vi "Autonomous Independent.vi"() -> ()   [LabVIEW 2015]
doc: "This VI is called when autonomous begins, and will automatically be terminated when autonomous ends. You can carry out timed or sensor driven robot movement independently without needing to return to the caller."
uses:
  <vilib>/Rock Robotics/WPI/Utilities/WPI_GetSetVariantRefNum.vi
  <vilib>/Rock Robotics/Network Tables/NT Write Numeric Array.vi
  <vilib>/Rock Robotics/Network Tables/NT Read Boolean.vi
  <vilib>/Rock Robotics/Network Tables/NT Write Boolean.vi
  <vilib>/Rock Robotics/Network Tables/NT Write Number.vi
  <vilib>/Rock Robotics/Network Tables/NT Read Number.vi
  <vilib>/Rock Robotics/WPI/RobotDrive/WPI_RobotDriveArcadeDrive_Standard(NoSaturation).vi
panel:
  out "Low Switch":bool
  out "High Switch":bool
  out "POT Sensor Meter":dbl(knob) scale=78.0..98.0
  out "POT Sensor Value":dbl
  # "Be sure to right-click and choose Data Operations>>Make Current Value default if you want to save the array values with the VI"
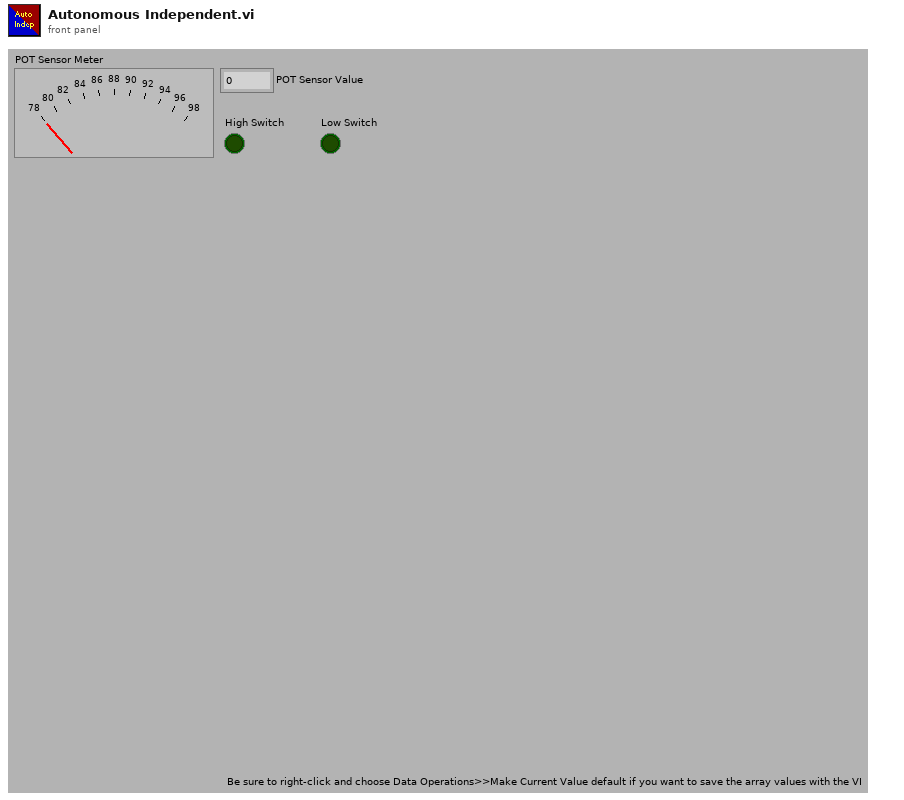
[diagram p1: front panel]
types:
  T1 = typedef "WPI_JoystickDevRef.ctl" = cluster{"Device":T2}
  T2 = typedef "WPI_JoystickDeviceEnum.ctl" = enum16{"USB 0", "USB 1", "USB 2", "USB 3", "USB 4", "USB 5"}
  T3 = typedef "WPI_SwitchDevRef.ctl" = cluster{"DevStatus":errorcluster, "DIO Channel":T4, "CntIndex":T5, "Normally Closed":bool}
  T4 = typedef "FPGA_DIOChannel.ctl" = enum8{"DIO 0", "DIO 1", "DIO 2", "DIO 3", "DIO 4", "DIO 5", "DIO 6", "DIO 7", "DIO 8", "DIO 9", "DIO MXP 0", "DIO MXP 1", "DIO MXP 2", "DIO MXP 3", "DIO MXP 4", "DIO MXP 5", "DIO MXP 6", "DIO MXP 7", "DIO MXP 8", "DIO MXP 9", "DIO MXP 10", "DIO MXP 11", "DIO MXP 12", "DIO MXP 13", "DIO MXP 14", "DIO MXP 15", "Invalid"}
  T5 = typedef "FPGA_CounterCtrSystemIndex.ctl" = enum8{"Ctr 0", "Ctr 1", "Ctr 2", "Ctr 3", "Ctr 4", "Ctr 5", "Ctr 6", "Ctr 7", "Invalid"}
  T6 = typedef "WPI_PotentiometerDevRef.ctl" = cluster{"DevStatus":errorcluster, "Analog Channel":T7, "Invert Output":bool}
  T7 = typedef "FPGA_AIChannel.ctl" = enum8{"AI 0", "AI 1", "AI 2", "AI 3", "AI MXP 0", "AI MXP 1", "AI MXP 2", "AI MXP 3", "Invalid"}
  T8 = typedef "WPI_MotorControlDeviceRef.ctl" = cluster{"DeviceStatus":errorcluster, "Type":T9, "PWM":cluster{"PWM Channel":T10, "DeadBand":T11}, "CAN":cluster{"Device Number":u8, "Control Mode":T12, "Semaphore":T13, "Max Vout":dbl, "TalonSRX Control Mode":T14}, "Invert":bool}
  T9 = typedef "WPI_MotorControlType.ctl" = enum16{"PWM", "CAN", "CANTalonSRX"}
  T10 = typedef "FPGA_DIOPWMChannel.ctl" = enum8{"PWM 0", "PWM 1", "PWM 2", "PWM 3", "PWM 4", "PWM 5", "PWM 6", "PWM 7", "PWM 8", "PWM 9", "PWM MXP 0", "PWM MXP 1", "PWM MXP 2", "PWM MXP 3", "PWM MXP 4", "PWM MXP 5", "PWM MXP 6", "PWM MXP 7", "PWM MXP 8", "PWM MXP 9", "Invalid"}
  T11 = typedef "WPI_PWMDeadband.ctl" = cluster{"Name":string, "maxPositivePwm":i32, "minPositivePwm":i32, "centerPwm":i32, "maxNegativePwm":i32, "minNegativePwm":i32, "angularRange":u16}
  T12 = typedef "WPI_CANJaguar_ControlMode.ctl" = enum8{"Percent VBus", "Current", "Speed", "Position", "Voltage"}
  T13 = typedef "Semaphore RefNum" = refnum<k1>
  T14 = typedef "WPI_CANTalonSRX_APIControlMode.ctl" = enum8{"Percent VBus", "Speed", "Position", "Slave", "Unchanged / Invalid", "Voltage Compensation", "Current", "Motion Profile"}
  T15 = typedef "WPI_RobotDriveDevRef.ctl" = cluster{"DevStatus":errorcluster, "Motors[]":T8[], "Square Inputs":bool, "Max Output":dbl}
  T16 = typedef "WPI_CounterDevRef.ctl" = cluster{"DevStatus":errorcluster, "CntIndex":T5}
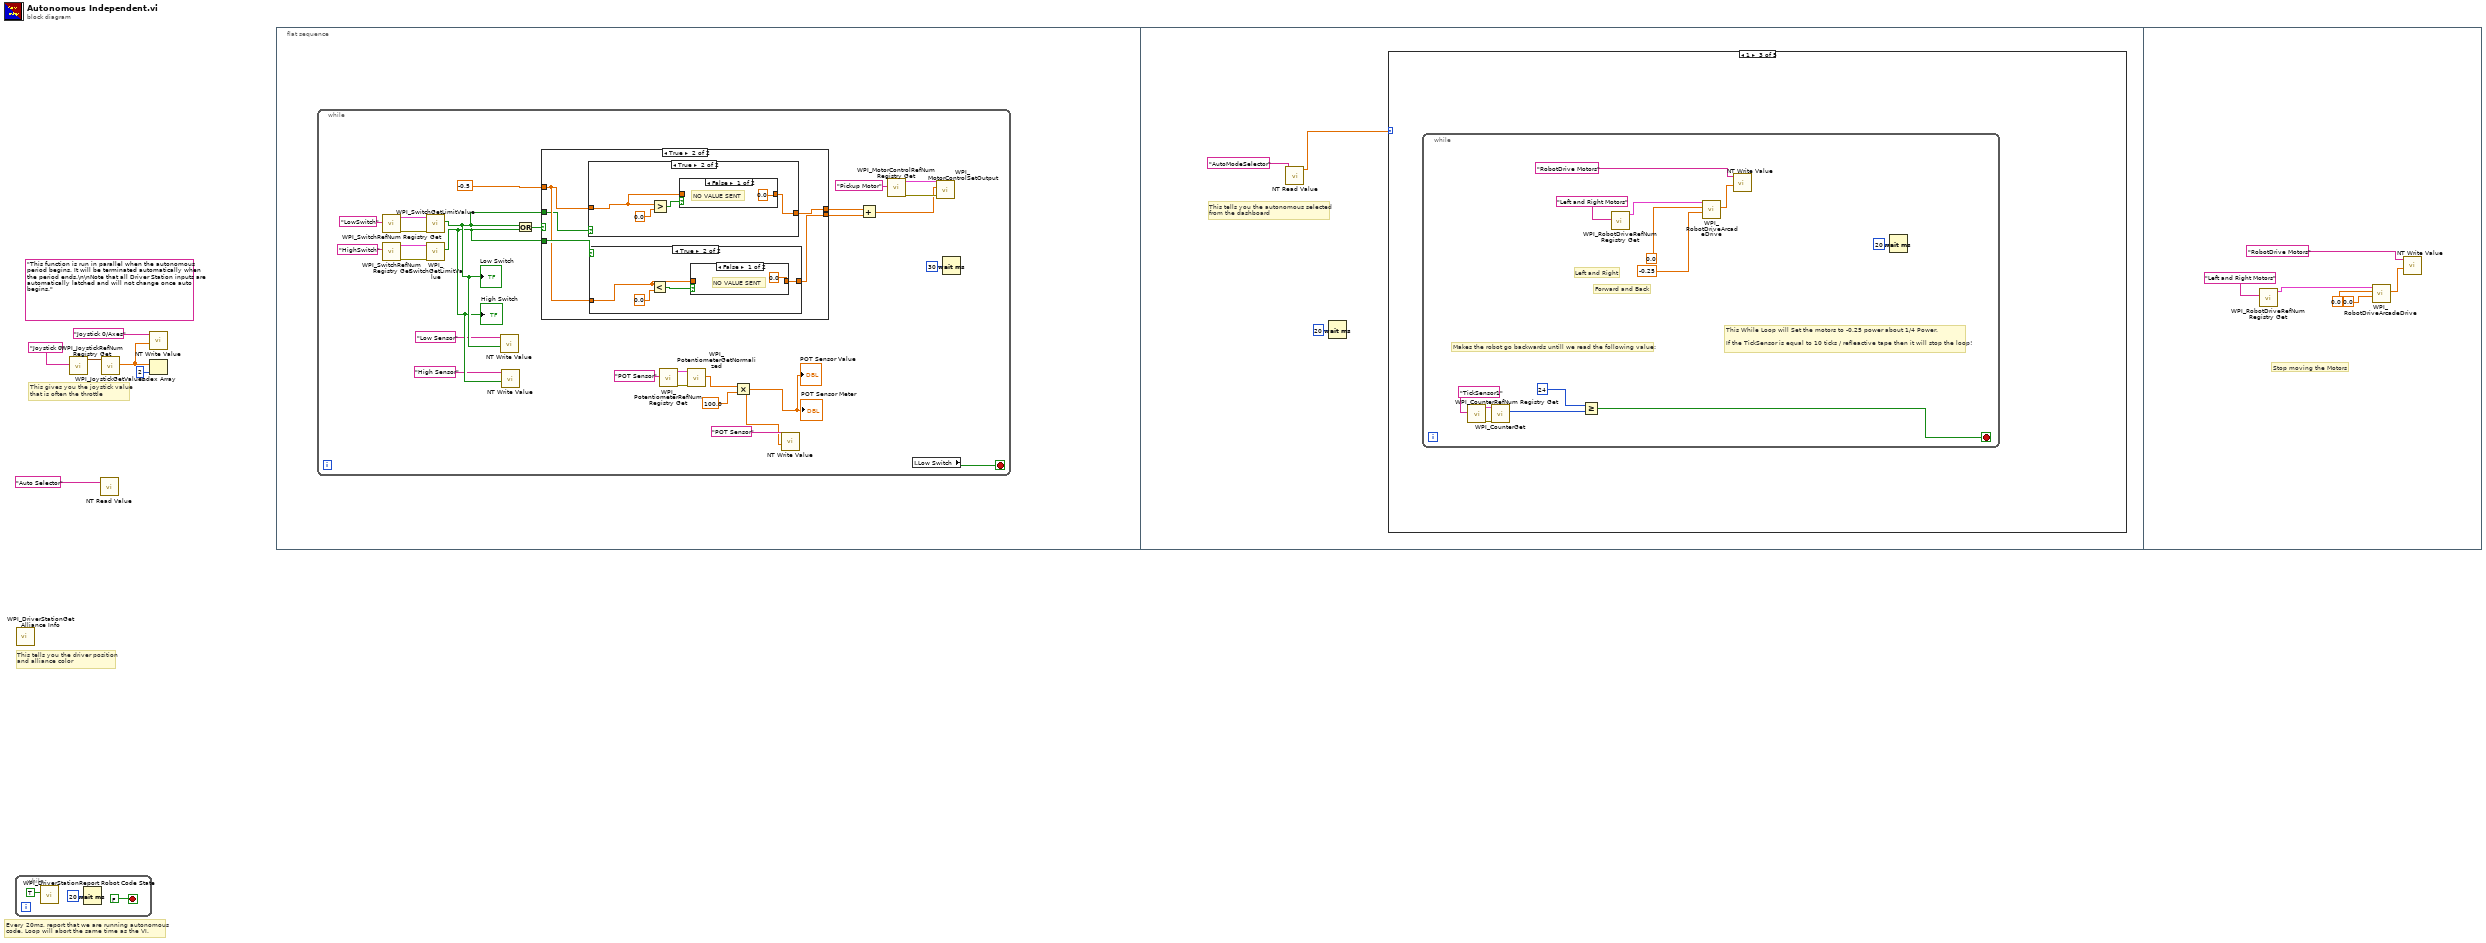
[diagram p0: block diagram]
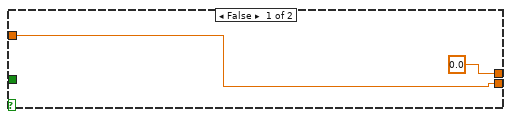
[diagram p2: hidden frame]
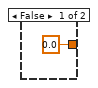
[diagram p3: hidden frame]
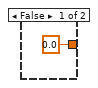
[diagram p5: hidden frame]
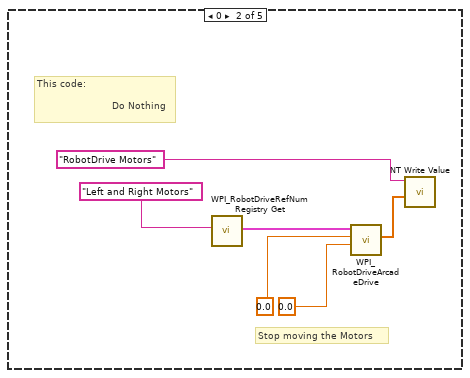
[diagram p8: hidden frame]
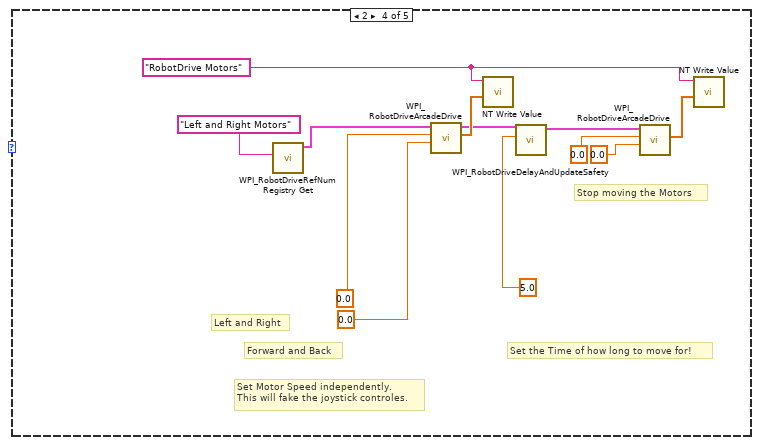
[diagram p9: hidden frame]
diagram:
  (unwired) "This function is run in parallel when the autonomous period begins. It will be terminated automatically when the period ends.\n\nNote that all Driver Station inputs are automatically latched and will not change once auto begins."
  # "Every 20ms, report that we are running autonomous\ncode. Loop will abort the same time as the VI."
  # "This gives you the joystick value\nthat is often the throttle"
  # "This tells you the driver position\nand alliance color"
  n1 = while {
    stop <- FALSE stop-if-true
    n2 = call <vilib>:"WPI_DriverStationReport Robot Code State.vi"("Autonomous"=TRUE) -> ()  [unwired: 10 in, 1 out]
    n3 = Wait (ms)(milliseconds to wait=u32 20) -> ()  [unwired: 1 out]
  }
  n4 = call <vilib>:"WPI_DriverStationGet Alliance Info.vi"() -> ()  [unwired: 12 out]
  n5 = call <vilib>:"WPI_JoystickRefNum Registry Get.vi"("refnum name"="Joystick 0") -> ("JoystickDevRef"=w5:T1)  [unwired: 1 in, 9 out]
  n6 = call-poly <vilib>:"NT Read Value.vi"("Name"="Auto Selector") -> ()  [unwired: 9 in, 2 out]
  n7 = call <vilib>:"WPI_JoystickGetValues.vi"("JoystickDevRef"=w5) -> ("Axes"=w3:dbl[])  [unwired: 6 in, 4 out]
  n8 = call-poly <vilib>:"NT Write Value.vi"("Numeric Array"=w3, "Name"="Joystick 0/Axes") -> ()  [unwired: 9 in, 1 out]
  n9 = Index Array(array=w3, index=2) -> ()  [unwired: 1 out]
  n10 = flat-sequence {
    frame #0 {
      n11 = while {
        stop <- w11 stop-if-true
        n12 = call <vilib>:"WPI_SwitchRefNum Registry Get.vi"("refnum name"="LowSwitch") -> ("error out"=w34:errorcluster, "SwitchDevRef"=w35:T3)  [unwired: 9 in]
        n13 = call <vilib>:"WPI_SwitchRefNum Registry Get.vi"("refnum name"="HighSwitch") -> ("error out"=w31:errorcluster, "SwitchDevRef"=w32:T3)  [unwired: 9 in]
        n14 = call <vilib>:"WPI_SwitchGetLimitValue.vi"("error in (no error)"=w34, "SwitchDevRef"=w35) -> ("Switch Pressed"=w19:bool)  [unwired: 7 in, 2 out]
        "Low Switch" <- w19
        n15 = call <vilib>:"WPI_SwitchGetLimitValue.vi"("error in (no error)"=w31, "SwitchDevRef"=w32) -> ("Switch Pressed"=w18:bool)  [unwired: 7 in, 2 out]
        "High Switch" <- w18
        n16 = call-poly <vilib>:"NT Write Value.vi"("Boolean"=w19, "Name"="Low Sensor") -> ()  [unwired: 9 in, 1 out]
        n17 = call-poly <vilib>:"NT Write Value.vi"("Boolean"=w18, "Name"="High Sensor") -> ()  [unwired: 9 in, 1 out]
        n18 = Or(x=w19, y=w18) -> (x .or. y?=w36:bool)
        n19 = case shown="True" w36 {
          tunnel: w19 -> [_ w41]
          tunnel: w18 -> [_ w43]
          tunnel: -0.5 ("Axes[1]") -> [w37 w42]
          tunnel: [0.0 ("Axes[1]") w40] -> w25
          tunnel: [w37 w39] -> w24
          frame False {
          }
          frame True {
            n20 = case shown="True" w41 {
              tunnel: w42 -> [_ w53]
              tunnel: [0.0 ("Axes[1]") w52] -> w40
              frame False {
              }
              frame True {
                n21 = Greater?(x=w53, y=0.0) -> (0:w54:bool)
                n22 = case shown="False" w54 {
                  tunnel: [0.0 ("Axes[1]") w57] -> w52
                  tunnel: w53 -> [_ w57]
                  frame False {
                    # "NO VALUE SENT"
                  }
                  frame True {
                  }
                }
              }
            }
            n23 = case shown="True" w43 {
              tunnel: w42 -> [_ w45]
              tunnel: [0.0 ("Axes[1]") w46] -> w39
              frame False {
              }
              frame True {
                n24 = Less?(x=w45, y=0.0) -> (x < y?=w47:bool)
                n25 = case shown="False" w47 {
                  tunnel: [0.0 ("Axes[1]") w50] -> w46
                  tunnel: w45 -> [_ w50]
                  frame False {
                    # "NO VALUE SENT"
                  }
                  frame True {
                  }
                }
              }
            }
          }
        }
        n26 = call <vilib>:"WPI_PotentiometerRefNum Registry Get.vi"("refnum name"="POT Sensor") -> ("error out"=w23:errorcluster, "PotDevRef"=w22:T6)  [unwired: 9 in]
        n27 = call <vilib>:"WPI_PotentiometerGetNormalized.vi"("error in"=w23, "PotDevRef"=w22) -> ("Normalized Value"=w15:dbl)  [unwired: 7 in, 2 out]
        n28 = Multiply(x=w15, y=100.0) -> (x*y=w13:dbl)
        "POT Sensor Value" <- w13
        "POT Sensor Meter" <- w13
        n29 = call-poly <vilib>:"NT Write Value.vi"("Numeric"=w13, "Name"="POT Sensor") -> ()  [unwired: 9 in, 1 out]
        n30 = Add(x=w25, y=w24) -> (x+y=w26:dbl)
        n31 = call <vilib>:"WPI_MotorControlRefNum Registry Get.vi"("refnum name"="Pickup Motor") -> ("error out"=w29:errorcluster, "MotorControlDevRef"=w28:T8)  [unwired: 9 in]
        n32 = local read "Low Switch"() -> (w11:bool)
        n33 = call <vilib>:"WPI_MotorControlSetOutput.vi"("error in (no error)"=w29, "Output"=w26, "MotorControlDevRef"=w28) -> ()  [unwired: 6 in, 3 out]
        n34 = Wait (ms)(milliseconds to wait=u32 30) -> ()  [unwired: 1 out]
      }
    }
    frame #1 {
      # "This tells you the autonomous selected\nfrom the dashboard"
      n35 = call-poly <vilib>:"NT Read Value.vi"("Name"="AutoModeSelector") -> ("Numeric"=w59:dbl)  [unwired: 9 in, 1 out]
      n36 = Wait (ms)(milliseconds to wait=u32 20) -> ()  [unwired: 1 out]
      n37 = case shown="1" w59 {
        frame Default {
          # "You can put your main auto here, or you can right-click on the case and make any\nother frame be the default case."
          # "This is the frame that will execute if no selection is made, or if it is not recognized"
        }
        frame 0 {
          # "Stop moving the Motors"
          # "This code:\n                   \n                         Do Nothing"
          n38 = call <vilib>:"WPI_RobotDriveRefNum Registry Get.vi"("refnum name"="Left and Right Motors") -> ("RobotDriveDevRef"=w61:T15)  [unwired: 1 in, 9 out]
          n39 = call-poly <vilib>:"WPI_RobotDriveArcadeDrive.vi"("Y axis value"=0.0 ("X axis value"), "X axis value"=0.0, "RobotDriveDevRef"=w61) -> ("Motor Values"=w65:dbl[])  [unwired: 1 in, 7 out]
          n40 = call-poly <vilib>:"NT Write Value.vi"("Numeric Array"=w65, "Name"="RobotDrive Motors") -> ()  [unwired: 9 in, 1 out]
        }
        frame 1 {
          n41 = while {
            stop <- w74 stop-if-true
            # "Makes the robot go backwards untill we read the following value:"
            # "This While Loop will Set the motors to -0.25 power about 1/4 Power.\n\nIf the TickSensor is equal to 10 ticks / refleactive tape then it will stop the loop!"
            # "Forward and Back"
            # "Left and Right"
            n42 = call <vilib>:"WPI_CounterRefNum Registry Get.vi"("refnum name"="TickSensor1") -> ("error out"=w78:errorcluster, "CounterDevRef"=w77:T16)  [unwired: 9 in]
            n43 = call <vilib>:"WPI_CounterGet.vi"("error in (no error)"=w78, "CounterDevRef in"=w77) -> ("Value"=w76:i32)  [unwired: 4 in, 5 out]
            n44 = Greater Or Equal?(x=24, y=w76) -> (x >= y?=w74:bool)
            n45 = call <vilib>:"WPI_RobotDriveRefNum Registry Get.vi"("refnum name"="Left and Right Motors") -> ("RobotDriveDevRef"=w73:T15)  [unwired: 1 in, 9 out]
            n46 = call-poly <vilib>:"WPI_RobotDriveArcadeDrive.vi"("Y axis value"=-0.25 ("X axis value"), "X axis value"=0.0, "RobotDriveDevRef"=w73) -> ("Motor Values"=w71:dbl[])  [unwired: 1 in, 7 out]
            n47 = call-poly <vilib>:"NT Write Value.vi"("Numeric Array"=w71, "Name"="RobotDrive Motors") -> ()  [unwired: 9 in, 1 out]
            n48 = Wait (ms)(milliseconds to wait=u32 20) -> ()  [unwired: 1 out]
          }
        }
        frame 2 {
          w90 = "RobotDrive Motors" ("Name")
          # "Forward and Back"
          # "Left and Right"
          # "Set Motor Speed independently.\nThis will fake the joystick controles."
          # "Set the Time of how long to move for!"
          # "Stop moving the Motors"
          n49 = call <vilib>:"WPI_RobotDriveRefNum Registry Get.vi"("refnum name"="Left and Right Motors") -> ("RobotDriveDevRef"=w91:T15)  [unwired: 1 in, 9 out]
          n50 = call-poly <vilib>:"WPI_RobotDriveArcadeDrive.vi"("Y axis value"=0.0 ("X axis value"), "X axis value"=0.0, "RobotDriveDevRef"=w91) -> ("Motor Values"=w89:dbl[], "RobotDriveDevRef"=w83:T15)  [unwired: 1 in, 6 out]
          n51 = call-poly <vilib>:"NT Write Value.vi"("Numeric Array"=w89, "Name"=w90) -> ()  [unwired: 9 in, 1 out]
          n52 = call <vilib>:"WPI_RobotDriveDelayAndUpdateSafety.vi"("Delay (s)"=5.0, "RobotDriveDevRef"=w83) -> ("RobotDriveDevRef 2"=w82:T15)  [unwired: 8 in, 1 out]
          n53 = call-poly <vilib>:"WPI_RobotDriveArcadeDrive.vi"("Y axis value"=0.0 ("X axis value"), "X axis value"=0.0, "RobotDriveDevRef"=w82) -> ("Motor Values"=w88:dbl[])  [unwired: 1 in, 7 out]
          n54 = call-poly <vilib>:"NT Write Value.vi"("Numeric Array"=w88, "Name"=w90) -> ()  [unwired: 9 in, 1 out]
        }
        frame 3 {
        }
      }
    }
    frame #2 {
      # "Stop moving the Motors"
      n55 = call <vilib>:"WPI_RobotDriveRefNum Registry Get.vi"("refnum name"="Left and Right Motors") -> ("RobotDriveDevRef"=w92:T15)  [unwired: 1 in, 9 out]
      n56 = call-poly <vilib>:"WPI_RobotDriveArcadeDrive.vi"("Y axis value"=0.0 ("X axis value"), "X axis value"=0.0, "RobotDriveDevRef"=w92) -> ("Motor Values"=w94:dbl[])  [unwired: 1 in, 7 out]
      n57 = call-poly <vilib>:"NT Write Value.vi"("Numeric Array"=w94, "Name"="RobotDrive Motors") -> ()  [unwired: 9 in, 1 out]
    }
  }
